vi "Close_Instr.vi"(8 "error in (no error)":errorcluster caption="entrée d'erreur (pas d'erreur)", 11 "Class Instrument Multimeter en entrée":refnum<class "Class Instrument Spectrum_Analyser.lvclass">) -> (0 "error out":errorcluster caption="sortie d'erreur", 3 "Class Instrument Multimeter en sortie":refnum<class "Class Instrument Spectrum_Analyser.lvclass">)   [LabVIEW 2020, in "Library Instrument & Equipement.lvlib" / "Library Instruments.lvlib" / "Class Instrument Spectrum_Analyser.lvclass"]
uses:
  Class Instrument Spectrum_Analyser.lvclass
  Class Instrument Spectrum_Analyser.lvclass/Class Instrument Spectrum_Analyser.ctl
  Spectrum Analyser/Class Spectrum Analyser (Default)/Class Spectrum Analyser (Default).lvclass
  Instrument (Default)/Class Instrument (Default).lvclass
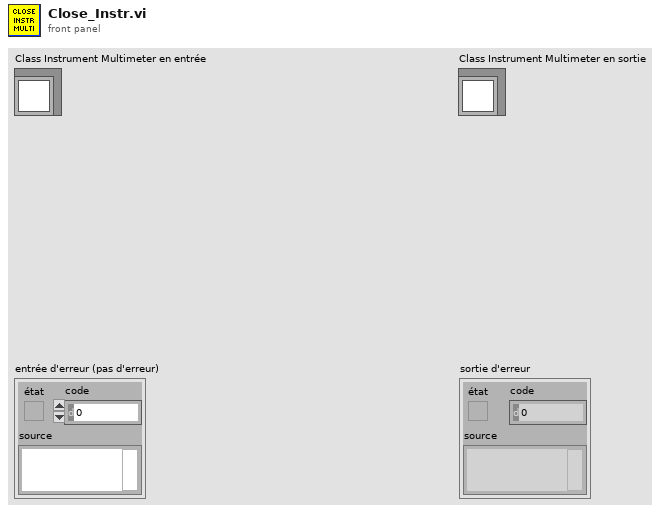
[diagram p1: front panel]
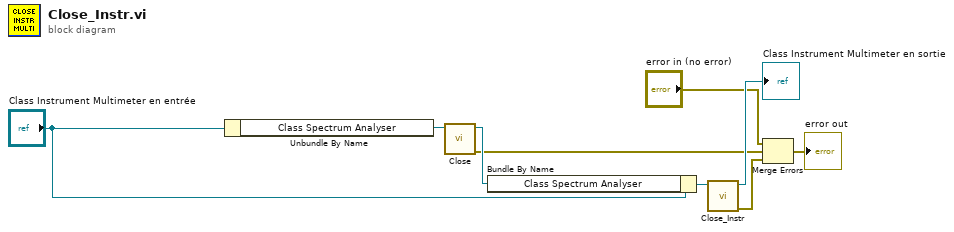
[diagram p0: block diagram]
diagram:
  n1 = Unbundle By Name("Class Instrument Multimeter en entrée") -> ("Class Spectrum Analyser"=w3:refnum<class "Class Spectrum Analyser (Default).lvclass">)
  n2 = call-dynamic "Close.vi"("Class Spectrum Analyser (Default) en entrée"=w3) -> ("error out"=w1:errorcluster, "Class Spectrum Analyser (Default) en sortie"=w2:refnum<class "Class Spectrum Analyser (Default).lvclass">)  [unwired: 9 in]
  n3 = Bundle By Name(cluster="Class Instrument Multimeter en entrée", "Class Spectrum Analyser"=w2) -> (w7:refnum<class "Class Instrument Spectrum_Analyser.lvclass">)
  n4 = call-parent "Close_Instr.vi"("Class Instrument (Default) en entrée"=w7) -> ("error out"=w5:errorcluster, "Class Instrument (Default) en sortie"=→"Class Instrument Multimeter en sortie":refnum<class "Class Instrument Spectrum_Analyser.lvclass">)  [unwired: 9 in]
  n5 = Merge Errors("error in (no error)", w1, w5) -> (→"error out":errorcluster)
